vi "IMU_read_RT_streaming_data.vi"() -> ()   [LabVIEW 2016]
doc: "This example demonstrates how to stream data from the FPGA target to the host PC using DMA FIFO."
uses:
  <vilib>/userdefined/Silver/nirio_resource_slv.ctl
  <vilib>/FPGAPlugInAG/cRIO-9116/niLvFpga_Open_cRIO-9116.vi
  <vilib>/rvi/interface/common/dynamic/niFpgaDynamicAddResources.vi
  <vilib>/Utility/error.llb/Error Cluster From Error Code.vi
  <vilib>/rvi/errors/niLvFpgaAdjustHostInterfaceError.vi
  <vilib>/FPGAPlugInAG/Dynamic/niLvFpga_Close_Dynamic.vi
  <vilib>/rvi/interface/nirviOpenFPGA/nirviOpenFPGA.xnode
  FPGA Bitfiles/IMUuse_FPGATarget_IMUreadFPGAstrea_DORLY4QJmyg.lvbitx
  IMU_read_FPGA_streaming_data.vi
  <vilib>/rvi/interface/nirviReadWriteControl/nirviReadWriteControl.xnode
  <vilib>/rvi/interface/nirviMethod/nirviMethod.xnode
  <vilib>/rvi/interface/nirviCloseFPGA/nirviCloseFPGA.xnode
  <vilib>/FPGAPlugInAG/Dynamic/niLvFpga_ReadFifo_Dynamic.vi
  <vilib>/rvi/errors/niLvFpgaMergeErrorWithErrorCode.vi
  NiFpgaLv.dll
  <vilib>/rvi/interface/Simulation/niFpgaSimulationCallBeginRW.vi
panel:
  out "Angular Rate (degree/s)":cluster{ext, ext, ext}(graph)
  in  "停止按钮":bool
  in  "波特率":T1(ring)=enum."460.8 kbps"
  in  "RIO Device":T2="RIO0"
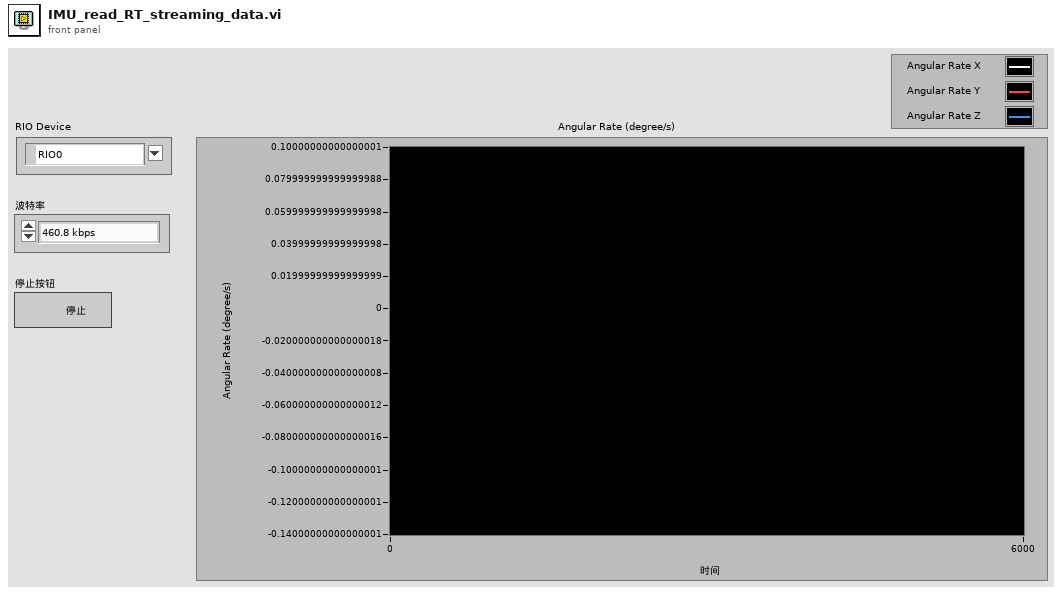
[diagram p1: front panel]
types:
  T1 = enum16{"75 bps", "110 bps", "134 bps", "150 bps", "300 bps", "600 bps", "1200 bps", "1800 bps", "2400 bps", "4800 bps", "7200 bps", "9600 bps", "14.4 kbps", "19.2 kbps", "28.8 kbps", "38.4 kbps", "57.6 kbps", "115.2 kbps", "230.4 kbps", "460.8 kbps", "921.6 kbps"}
  T2 = typedef "nirio_resource_slv.ctl" = tag
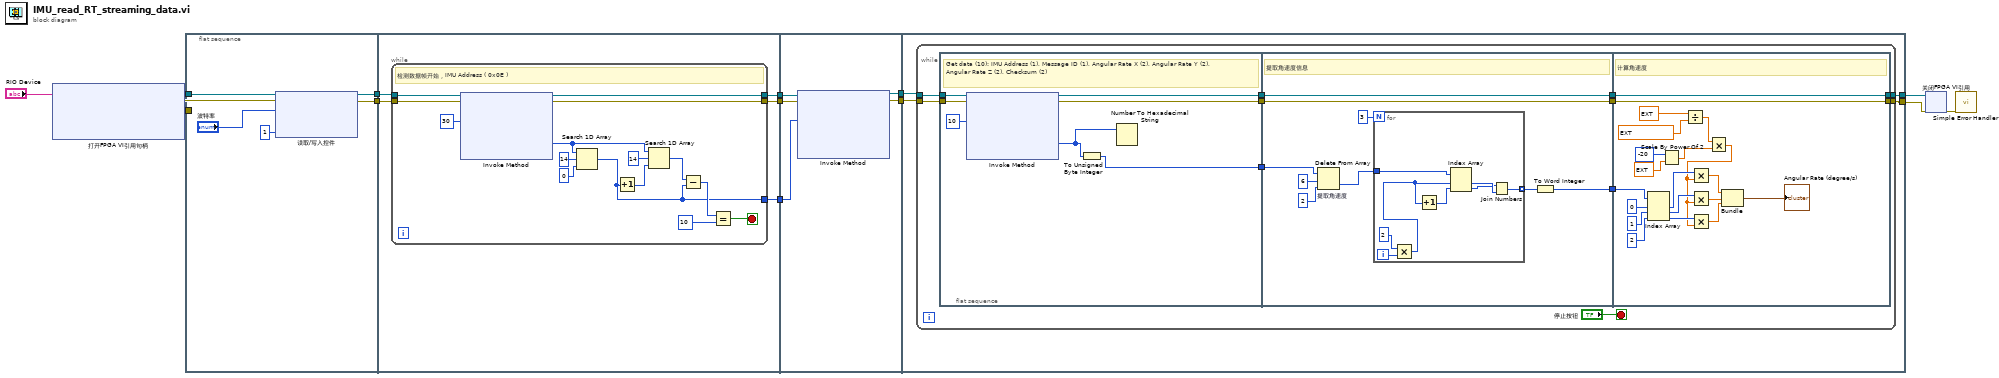
[diagram p0: block diagram]
diagram:
  n1 = xnode "打开FPGA VI引用句柄"("资源名称"="RIO Device") -> ("FPGA VI引用输出"=w12:refnum<k20>, "错误输出"=w11:errorcluster)  [unwired: 1 in]
  n2 = flat-sequence {
    tunnel: w12 -> [w19]
    tunnel: w11 -> [w18]
    tunnel: [w17] -> w9
    tunnel: [w16] -> w8
    tunnel: w9 -> [w24]
    tunnel: w8 -> [w23]
    tunnel: [w22] -> w7
    tunnel: [w21] -> w6
    tunnel: [w20] -> w5
    tunnel: w7 -> [w44]
    tunnel: w6 -> [w43]
    tunnel: w5 -> [w42]
    tunnel: [w41] -> w4
    tunnel: [w40] -> w3
    tunnel: w4 -> [w48]
    tunnel: w3 -> [w47]
    tunnel: [w46] -> w2
    tunnel: [w45] -> w1
    frame #0 {
      n3 = xnode "读取/写入控件"("FPGA VI引用输入"=w19, "错误输入"=w18, "波特率"="波特率", "Number of bytes"=u16 1) -> ("FPGA VI引用输出"=w17:refnum<k20>, "错误输出"=w16:errorcluster)  [unwired: 1 out]
    }
    frame #1 {
      n4 = while "While循环" {
        tunnel: w23 -> [w38]
        tunnel: [w36] -> w21
        tunnel: w24 -> [w39]
        tunnel: [w37] -> w22
        tunnel: [w25] -> w20
        stop <- w26 stop-if-true
        # "检测数据帧开始，IMU Address ( 0x0E )"
        n5 = xnode "Invoke Method"("FPGA VI引用输入"=w39, "错误输入"=w38, "元素数量"=u32 30) -> ("FPGA VI引用输出"=w37:refnum<k20>, "错误输出"=w36:errorcluster, "数据"=w31:i16[])  [unwired: 1 in, 1 out]
        n6 = Search 1D Array(1D array=w31, element=i16 14 ("IMU Address"), start index (0)=0 ("开始索引(0)")) -> (index of element=w25:i32)
        n7 = Increment(x=w25) -> (x+1=w33:i32)
        n8 = Search 1D Array(1D array=w31, element=i16 14 ("IMU Address"), start index (0)=w33) -> (index of element=w32:i32)
        n9 = Subtract(x=w32, y=w25) -> (x-y=w29:i32)
        n10 = Equal?(x=w29, y=10) -> (x = y?=w26:bool)
      }
    }
    frame #2 {
      n11 = xnode "Invoke Method"("FPGA VI引用输入"=w44, "错误输入"=w43, "元素数量"=w42) -> ("FPGA VI引用输出"=w41:refnum<k20>, "错误输出"=w40:errorcluster)  [unwired: 1 in, 2 out]
    }
    frame #3 {
      n12 = while {
        tunnel: w47 -> [w58]
        tunnel: [w56] -> w45
        tunnel: w48 -> [w59]
        tunnel: [w57] -> w46
        stop <- "停止按钮" stop-if-true
        n13 = flat-sequence "平铺式顺序结构" {
          tunnel: w59 -> [w66]
          tunnel: w58 -> [w65]
          tunnel: [w64] -> w54
          tunnel: [w63] -> w53
          tunnel: [w60] -> w52
          tunnel: w54 -> [w75]
          tunnel: w53 -> [w74]
          tunnel: w52 -> [w69]
          tunnel: [w75] -> w51
          tunnel: [w74] -> w50
          tunnel: [w67] -> w49
          tunnel: [w102] -> w56
          tunnel: [w103] -> w57
          tunnel: w51 -> [w103]
          tunnel: w50 -> [w102]
          tunnel: w49 -> [w94]
          frame #0 {
            # "Get data (10): IMU Address (1), Message ID (1), Angular Rate X (2), Angular Rate Y (2), Angular Rate Z (2), Checksum (2)"
            n14 = xnode "Invoke Method"("FPGA VI引用输入"=w66, "错误输入"=w65, "元素数量"=u32 10) -> ("FPGA VI引用输出"=w64:refnum<k20>, "错误输出"=w63:errorcluster, "数据"=w61:i16[])  [unwired: 1 in, 1 out]
            n15 = To Unsigned Byte Integer(number=w61) -> (unsigned 8bit integer=w60:u8[])
            n16 = Number To Hexadecimal String(2:w61) -> ()  [unwired: 1 in, 1 out]
          }
          frame #1 {
            # "提取角速度信息"
            n17 = Delete From Array "提取角速度"(array=w69, length=6 ("数据域长度"), index=2 ("角速度数据开始位置")) -> (deleted portion=w70:u8[])  [unwired: 1 out]
            n18 = for {
              N: 3 -> [_]
              tunnel: w70 -> [w80]
              tunnel: [w77] -> w68 mode=indexing
              i -> [w83]
              n19 = Multiply(x=2, y=w83) -> (x*y=w76:i32)
              n20 = Increment(x=w76) -> (x+1=w81:i32)
              n21 = Index Array(array=w80, index #1=w76, index #2=w81) -> (element #1=w79:u8, element #2=w78:u8)
              n22 = Join Numbers(hi=w78, lo=w79) -> ((hi.lo)=w77:u16)
            }
            n23 = To Word Integer(number=w68) -> (16bit integer=w67:i16[])
          }
          frame #2 {
            # "计算角速度"
            n24 = Index Array(array=w94, index #1=0 ("索引"), index #2=1 ("索引"), index #3=2 ("索引")) -> (element #1=w92:i16, element #2=w91:i16, element #3=w93:i16)
            n25 = Scale By Power Of 2 ("按2的幂缩放")(n=i16 -20, x=ext 600.0) -> (x*2^n=w87:ext)
            n26 = Divide(x=ext 180.0 ("y"), y=ext 3.141592653) -> (x/y=w88:ext)
            n27 = Multiply(x=w88, y=w87) -> (x*y=w86:ext)
            n28 = Multiply(x=w92, y=w86) -> (x*y=w101:ext)
            n29 = Multiply(x=w91, y=w86) -> (x*y=w100:ext)
            n30 = Multiply(x=w93, y=w86) -> (x*y=w85:ext)
            n31 = Bundle(w101, w100, w85) -> (→"Angular Rate (degree/s)":cluster{ext, ext, ext})  [unwired: 1 in]
          }
        }
      }
    }
  }
  n32 = xnode "关闭FPGA VI引用"("FPGA VI引用输入"=w2, "错误输入"=w1) -> ("错误输出"=w10:errorcluster)
  n33 = call <vilib>:"Simple Error Handler.vi"("error in (no error)"=w10) -> ()  [unwired: 4 in, 5 out]
